vi "mod_PM CE Demodulation (block processing).vi"(6 "carrier correction?":bool, 7 "weighting window":T1(ring)=enum."Hanning", 8 "kp":dbl format="%.2p", 9 "reset?":bool, 10 "fs":dbl format="%.2p", 11 "x":cdb[](array[numeric]) format="%.2f") -> (0 "carrier phase [rad]":dbl format="%.2f", 1 "carrier frequency":dbl format="%.2f", 3 "PM demod":dbl[](array[numeric]) format="%.2f")   [LabVIEW 2020, in "niAMT.lvlib"]
doc: "This VI performs PM demodulation for incoming analog I-Q signal. Basically the input signal is the base band I-Q signal with possible some carrier offset. If the carrier correction boolean is on, this VI will perform weighted linear fit to estimate the carrier frequency and phase. The weighting function can be chosen from a variety of window functions. The estimated value will be returned as carrier frequency in hertz and carrier phase in radian. If the boolean is off, those two values will be set to zero."
uses:
  <vilib>/addons/Modulation/niAMT.lvlib
  <vilib>/Analysis/0measdsp.llb/Scaled Time Domain Window (DBL).vi
  <vilib>/Analysis/NI_AALPro.lvlib
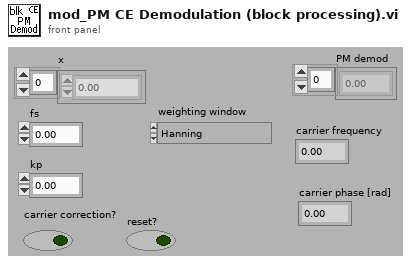
[diagram p1: front panel]
types:
  T1 = enum16{"None ", "Hanning", "Hamming", "Blackman-Harris", "Exact Blackman", "Blackman", "Flat Top", "4 Term B-Harris ", "7 Term B-Harris", "Low Sidelobe"}
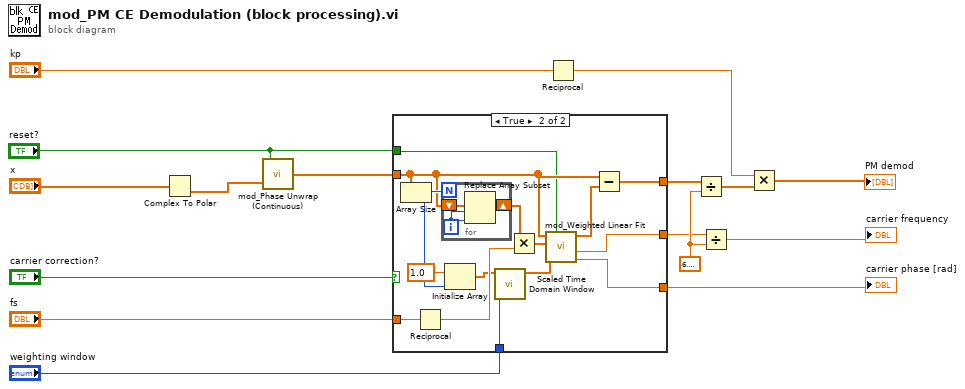
[diagram p0: block diagram]
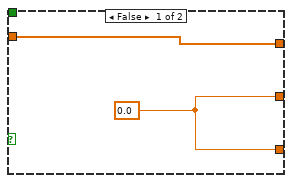
[diagram p2: hidden frame]
diagram:
  w8 = 6.283185307179586
  n1 = Complex To Polar(r * e^(i*theta)="x") -> (theta=w4:dbl[])  [unwired: 1 out]
  n2 = call <vilib>:"mod_Phase Unwrap (Continuous).vi"("Input Signal"=w4, "Reset"="reset?") -> ("Phase Unwrapped"=w3:dbl[])
  n3 = case shown="True" "carrier correction?" {
    tunnel: w3 -> [w17 w21]
    tunnel: "fs" -> [_ w33]
    tunnel: [w18 w28] -> w7
    tunnel: [w17 w27] -> w2
    tunnel: [w18 w29] -> w13
    tunnel: "weighting window" -> [_ w26]
    tunnel: "reset?" -> [_ w19]
    frame False {
      w18 = 0.0 ("slope")
    }
    frame True {
      n4 = Array Size(array=w21) -> (size(s)=w25:i32)
      n5 = Reciprocal(x=w33) -> (1/x=w32:dbl)
      n6 = for {
        N: w25 -> [_]
        shift-right: [w35] -> w22
        shift-left: w21 -> [w34]
        i -> [w36]
        n7 = Replace Array Subset(array=w34, new element=w36, index=w36) -> (w35:dbl[])
      }
      n8 = Initialize Array(1.0 ("element"), w25) -> (w23:dbl[])
      n9 = call-poly <vilib>:"Scaled Time Domain Window.vi"("window"=w26, "X"=w23) -> ("Windowed X"=w20:dbl[])  [unwired: 1 in, 8 out]
      n10 = Multiply(x=w22, y=w32) -> (x*y=w31:dbl[])
      n11 = call <vilib>:"mod_Weighted Linear Fit.vi"("reset?"=w19, "weights"=w20, "X Values"=w31, "Y Values"=w21) -> ("intercept"=w29:dbl, "slope"=w28:dbl, "weighted linear fit"=w30:dbl[])  [unwired: 5 out]
      n12 = Subtract(x=w21, y=w30) -> (x-y=w27:dbl[])
    }
  }
  "carrier phase [rad]" <- w13
  n13 = Reciprocal(x="kp") -> (1/x=w5:dbl)
  n14 = Divide(x=w2, y=w8) -> (x/y=w6:dbl[])
  n15 = Divide(x=w7, y=w8) -> (x/y=→"carrier frequency":dbl)
  n16 = Multiply(x=w5, y=w6) -> (x*y=→"PM demod":dbl[])
